vi "Test VISA GPS.vi"() -> ()   [LabVIEW 2012]
uses:
  nmea/VISA GPS/VISA GPS.lvclass
  nmea/nmea/nmea.lvclass
  nmea/nmea/Fix.ctl
  nmea/nmea/Velocity.ctl
  nmea/nmea/DOP.ctl
  nmea/nmea/Satellite.ctl
  nmea/nmea/Fix Type.ctl
  nmea/nmea/Fix Mode.ctl
  nmea/nmea/Full Data.ctl
panel:
  in  "Stop":bool
  out "Full Data":T1 {"Fix"."Longitude" format="%_16f"; "Fix"."Latitude" format="%_16f"}
  # "PRN"
  # "Chan"
  # "Elev"
  # "Az"
  # "SnR"
  # "Used"
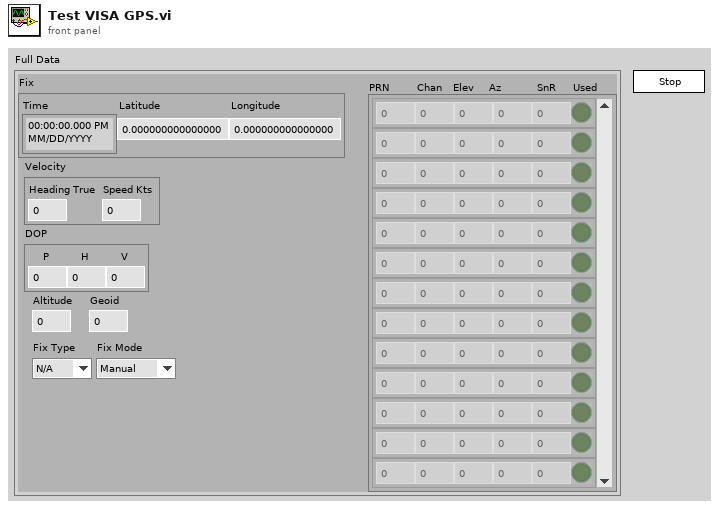
[diagram p1: front panel]
types:
  T1 = typedef "nmea.lvlib/nmea.lvclass/Full Data.ctl" = cluster{"Fix":T2, "Velocity":T3, "DOP":T4, "Altitude":dbl, "Geoid":dbl, "Satellites":T5[], "Fix Type":T6, "Fix Mode":T7}
  T2 = typedef "nmea.lvlib/nmea.lvclass/Fix.ctl" = cluster{"Time":timestamp, "Latitude":dbl, "Longitude":dbl}
  T3 = typedef "nmea.lvlib/nmea.lvclass/Velocity.ctl" = cluster{"Heading True":dbl, "Speed Kts":dbl}
  T4 = typedef "nmea.lvlib/nmea.lvclass/DOP.ctl" = cluster{"P":dbl, "H":dbl, "V":dbl}
  T5 = typedef "nmea.lvlib/nmea.lvclass/Satellite.ctl" = cluster{"PRN":u8, "Channel":u8, "Elevation":u8, "Azimuth":u16, "SNR":u8, "Active":bool}
  T6 = typedef "nmea.lvlib/nmea.lvclass/Fix Type.ctl" = enum16{"N/A", "None", "2D", "3D"}
  T7 = typedef "nmea.lvlib/nmea.lvclass/Fix Mode.ctl" = enum16{"Manual", "Auto 2/3D"}
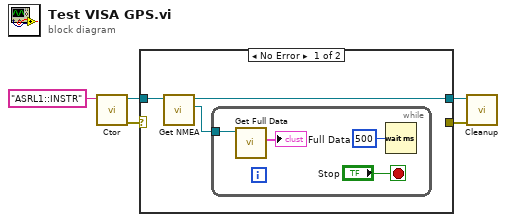
[diagram p0: block diagram]
diagram:
  n1 = call "Ctor.vi"("VISA Port"="ASRL1::INSTR") -> ("error out"=w3:errorcluster, "VISA GPS out"=w4:refnum<class "VISA GPS.lvclass">)  [unwired: 9 in]
  n2 = case shown="No Error" w3 {
    selector: w3 -> [_ w13]
    tunnel: w4 -> [w8 w14]
    tunnel: [w6 w14] -> w2
    tunnel: [_ w13] -> w1
    frame No Error {
      n3 = call "Get NMEA.vi"("VISA GPS in"=w8) -> ("NMEA"=w7:refnum<class "nmea.lvclass">, "VISA GPS out"=w6:refnum<class "VISA GPS.lvclass">)  [unwired: 8 in, 1 out]
      n4 = while {
        tunnel: w7 -> [w10]
        stop <- "Stop" stop-if-true
        n5 = call "Get Full Data.vi"("nmea in"=w10) -> ("Full Data"=→"Full Data":T1)  [unwired: 8 in, 2 out]
        n6 = Wait (ms)(milliseconds to wait=u32 500) -> ()  [unwired: 1 out]
      }
    }
    frame Error {
    }
  }
  n7 = call "Cleanup.vi"("error in (no error)"=w1, "VISA GPS in"=w2) -> ()  [unwired: 9 in, 1 out]
